vi "CalculateCoordinatesinArrayformforResavingData_171213.vi"(0 "X1":sgl[](array[numeric]), 1 "Y1":sgl[](array[numeric]), 2 "X2":sgl[](array[numeric]), 3 "Y2":sgl[](array[numeric])) -> (9 "X1-X2":sgl[](array[numeric]), 11 "Y1-Y2":sgl[](array[numeric]), 14 "sin(a)":sgl[](array[numeric]), 15 "R from center":sgl[](array[numeric]), 16 "Mouse Xc":sgl[](array[numeric]), 17 "Mouse Yc":sgl[](array[numeric]), 18 "Cage Xc":sgl[](array[numeric]), 19 "Cage Yc":sgl[](array[numeric]))   [LabVIEW 2016]
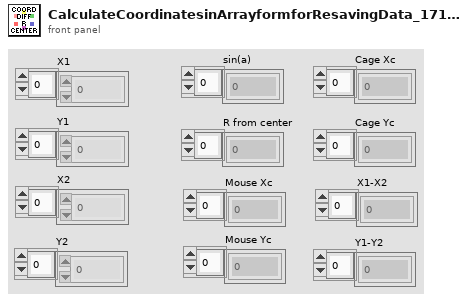
[diagram p1: front panel]
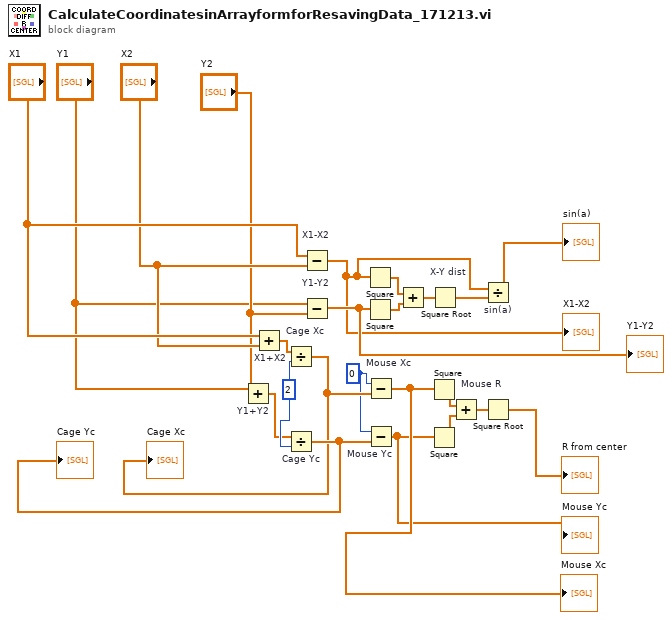
[diagram p0: block diagram]
diagram:
  w1 = 0
  w4 = 2
  n1 = Add "Y1+Y2"(x="Y1", y="Y2") -> (x+y=w3:sgl[])
  n2 = Add "X1+X2"(x="X1", y="X2") -> (x+y=w2:sgl[])
  n3 = Divide "Cage Xc"(x=w2, y=w4) -> (x/y=w14:sgl[])
  "Cage Xc" <- w14
  n4 = Divide "Cage Yc"(x=w3, y=w4) -> (x/y=w15:sgl[])
  "Cage Yc" <- w15
  n5 = Subtract "X1-X2"(x="X1", y="X2") -> (x-y=w11:sgl[])
  "X1-X2" <- w11
  n6 = Subtract "Y1-Y2"(x="Y1", y="Y2") -> (x-y=w12:sgl[])
  "Y1-Y2" <- w12
  n7 = Square(x=w11) -> (x^2=w7:sgl[])
  n8 = Square(x=w12) -> (x^2=w8:sgl[])
  n9 = Subtract "Mouse Xc"(x=w1, y=w14) -> (x-y=w22:sgl[])
  "Mouse Xc" <- w22
  n10 = Subtract "Mouse Yc"(x=w1, y=w15) -> (x-y=w19:sgl[])
  "Mouse Yc" <- w19
  n11 = Add(x=w7, y=w8) -> (x+y=w9:sgl[])
  n12 = Square(x=w22) -> (x^2=w16:sgl[])
  n13 = Square(x=w19) -> (x^2=w17:sgl[])
  n14 = Square Root "X-Y dist"(x=w9) -> (sqrt(x)=w10:sgl[])
  n15 = Add(x=w16, y=w17) -> (x+y=w18:sgl[])
  n16 = Divide "sin(a)"(x=w11, y=w10) -> (x/y=→"sin(a)":sgl[])
  n17 = Square Root "Mouse R"(x=w18) -> (sqrt(x)=→"R from center":sgl[])
